vi "FPGA_fast cycles-5.vi"() -> ()   [LabVIEW 2013]
uses:
  FPGA_run-states.ctl
  <vilib>/rvi/Emulation/niFpgaSctlEmulationGetInTimedLoop.vi
  <vilib>/rvi/Emulation/niFpgaEmulationReportErrorSimple.vi
  <vilib>/rvi/Emulation/niFpgaGetClockAttributes.vi
  <vilib>/rvi/Emulation/niFpgaCriticalErrorInLSC.vi
  <vilib>/rvi/eio/common/nirviEmuTemplateMethod_errors.vi
  <vilib>/rvi/FIFO/Fifo_Resource/nirvififoEmulationReadFpgaImpl.vi
  <vilib>/rvi/DataTransferAndStorage/Container/Common/niFpgaContainerGetUniqueNameForEmu.vi
  <vilib>/rvi/Emulation/niFpgaProcessEmulError.vi
  <vilib>/rvi/Memory/Memory_Emulation/nirvimemoryEmulation.vi
  <vilib>/rvi/Memory/Memory_Emulation/nirvimemoryFastEmulation.vi
  <vilib>/rvi/Memory/Memory_Emulation/niFpgaMemoryEmulationCacheClearOnFirstRun.vi
  <vilib>/rvi/Memory/Memory_Emulation/nirvimemoryEmulationManagerCache_MakeExclusive.vi
  <vilib>/rvi/Memory/Memory_Emulation/niFpgaMemoryEmulationValidateCache.vi
  <vilib>/rvi/Memory/Memory_Emulation/nirvimemoryEmulationManagerCache_ReleaseExclusive.vi
  <vilib>/rvi/Memory/Memory_Emulation/nirvimemoryEmulationManagerCache_InsertValue.vi
  <vilib>/Utility/error.llb/Clear Errors.vi
  <vilib>/rvi/Memory/Memory_Emulation/nirvimemoryEmulationManagerCache_SetValue.vi
  <vilib>/rvi/Emulation/niFpgaSctlEmulationResourceMgr.vi
  <vilib>/rvi/Memory/Memory_Emulation/nirvimemoryEmulationManagerCache_GetValue.vi
  <vilib>/rvi/Memory/Memory_Emulation/nirvimemoryFastEmulationFpgaImpl.vi
  <instcachedir>/0/nirvimemoryFastEmulationFpgaImpl_5FBAB50466BC4C939F684F8805638BFC.lvgen/nirvimemoryFastEmulationFpgaImpl_5FBAB50466BC4C939F684F8805638BFC_004.vi
  <vilib>/rvi/FIFO/Fifo_Resource/nirvififoEmulationWriteFpgaImpl.vi
  <vilib>/eio/EIONode/EIONode.xnode
  <vilib>/rvi/DataTransferAndStorage/Container/XNode/niFpgaContainer.xnode
  <vilib>/rvi/FIFO/Fifo_Resource/nirvififoEmulationRead.vi
  <vilib>/rvi/FIFO/Fifo_Resource/nirvififoEmulationWrite.vi
panel:
  in  "start ind":u32
  out "stopped":bool=TRUE
  out "ramp":bool
  out "trigDAC":bool
  in  "order in":u64=360850920143060992
  in  "get order":bool
  in  "trig dur (us)":u16=100
  in  "us per DAC":u32=1000
  out "gen trig":bool
  in  "Stop seq":bool=TRUE
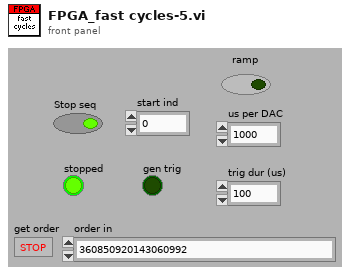
[diagram p1: front panel]
types:
  T1 = typedef "FPGA_run-states.ctl" = enum16{"stopped", "check", "reserve", "run", "release"}
  T2 = cluster{"Boolean array[0]":bool, "Boolean array[1]":bool, "Boolean array[2]":bool, "Boolean array[3]":bool, "Boolean array[4]":bool, "Boolean array[5]":bool, "Boolean array[6]":bool, "Boolean array[7]":bool, "Boolean array[8]":bool, "Boolean array[9]":bool}
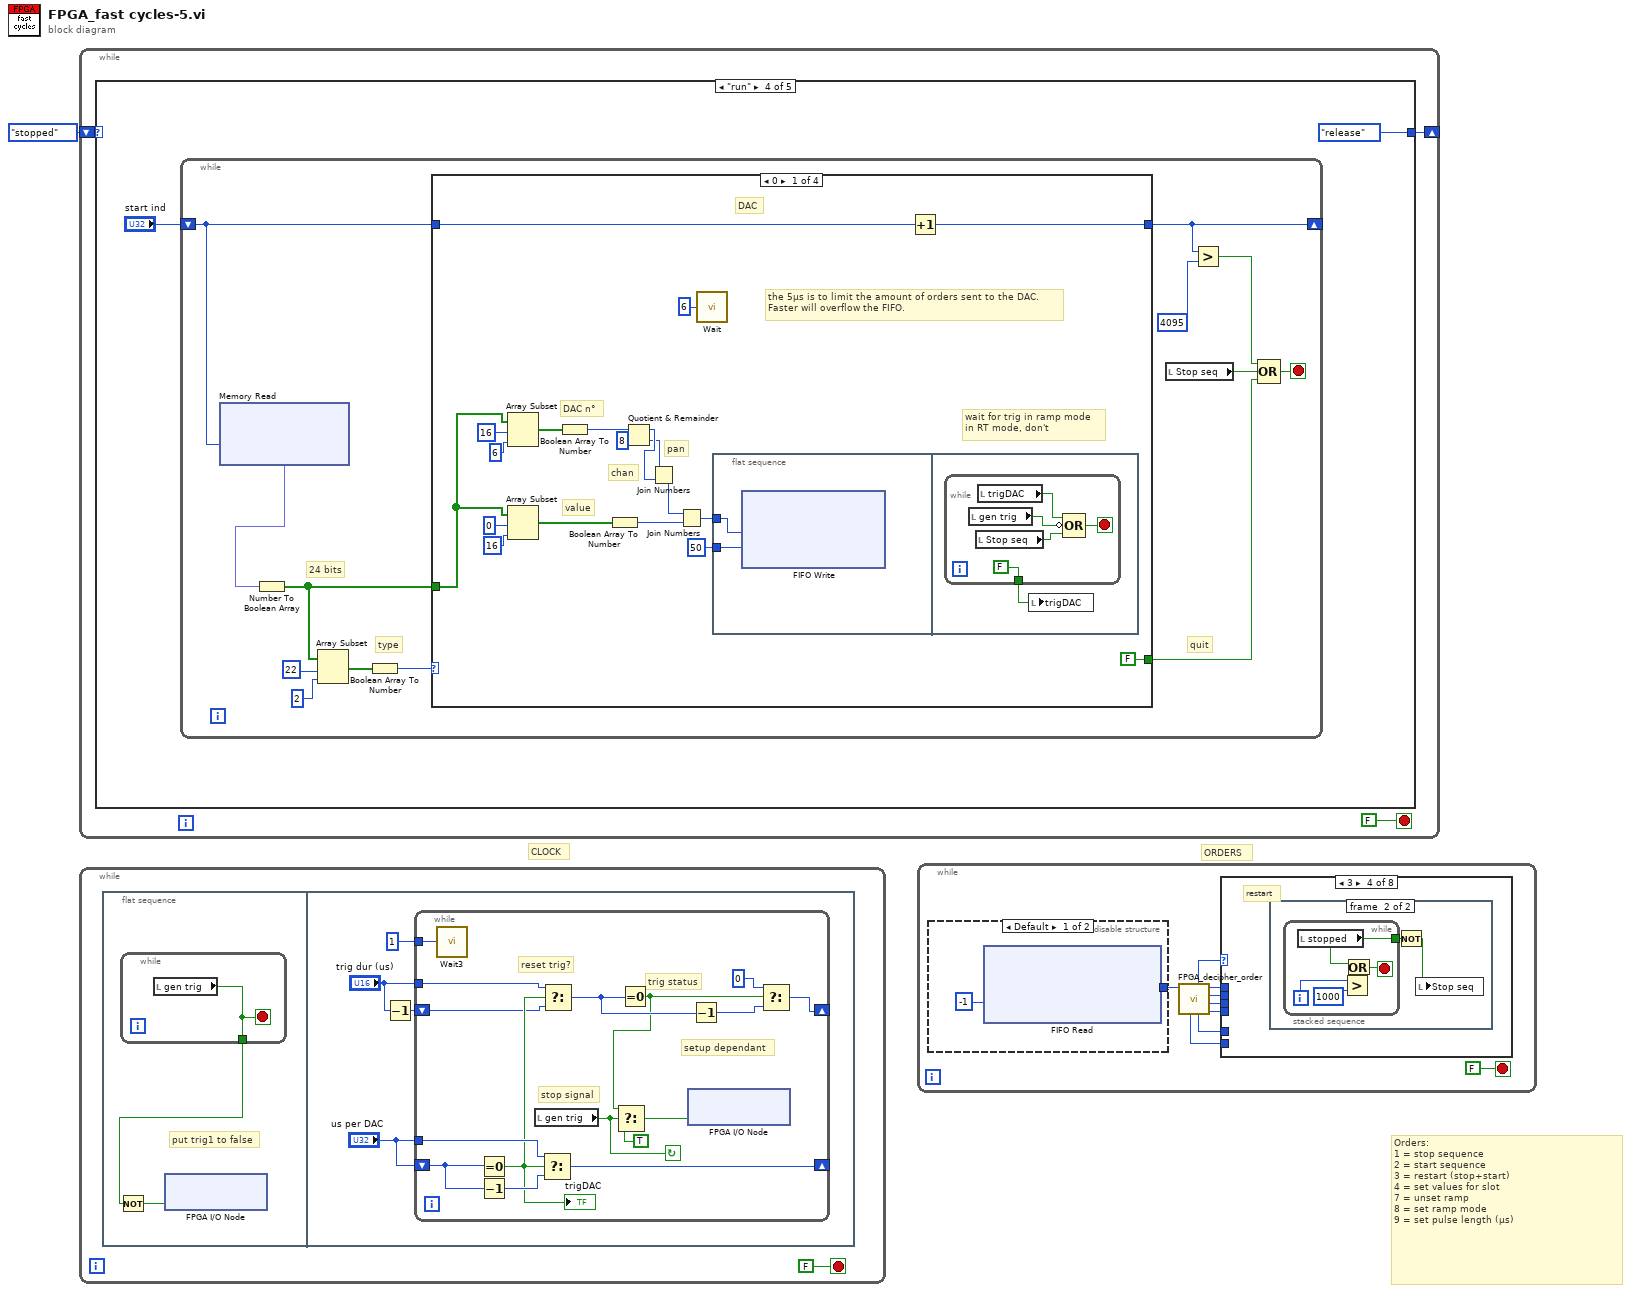
[diagram p0: block diagram]
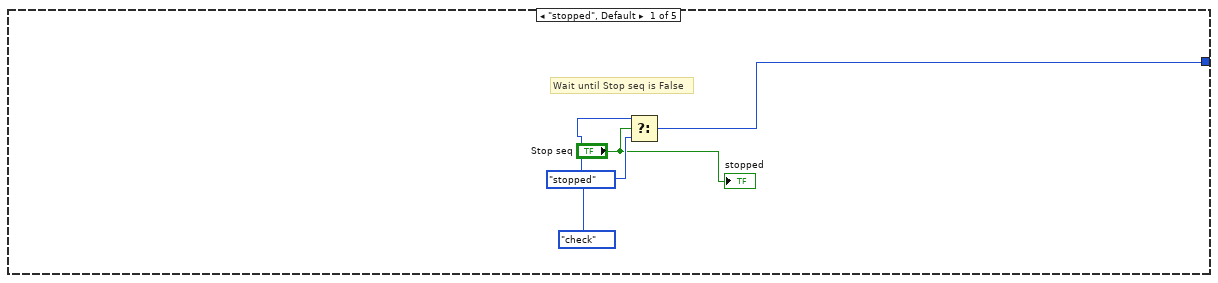
[diagram p2: hidden frame]
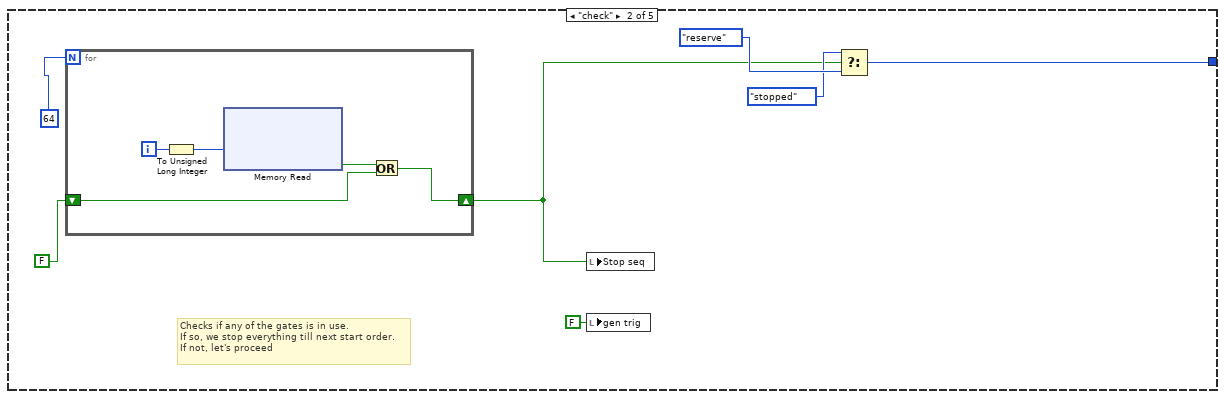
[diagram p3: hidden frame]
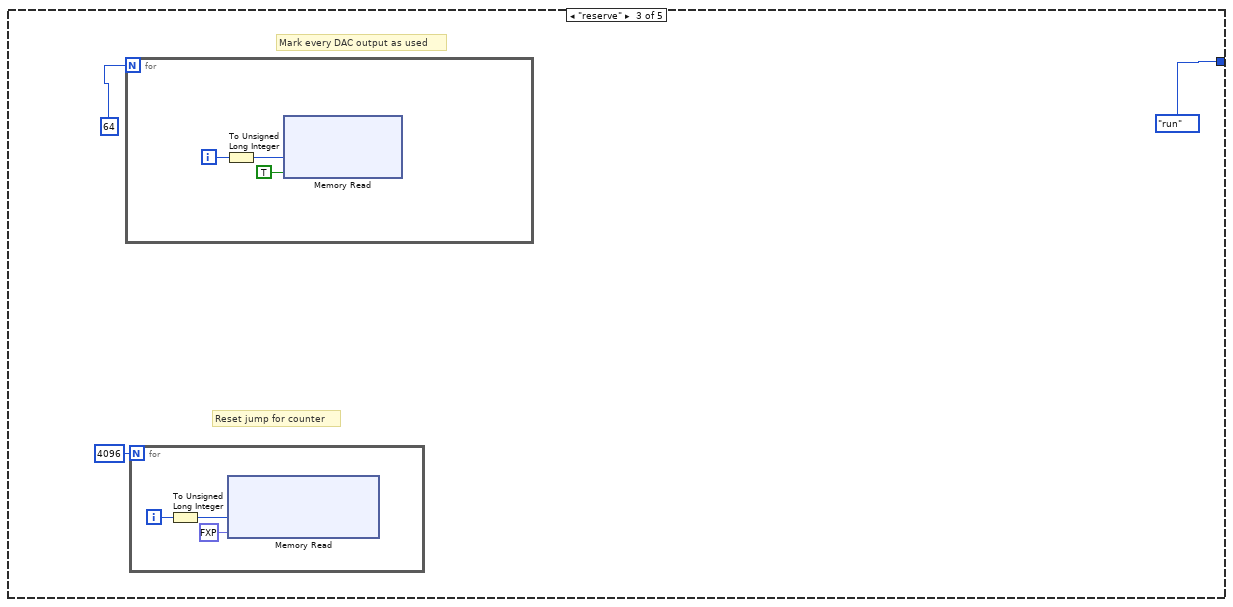
[diagram p4: hidden frame]
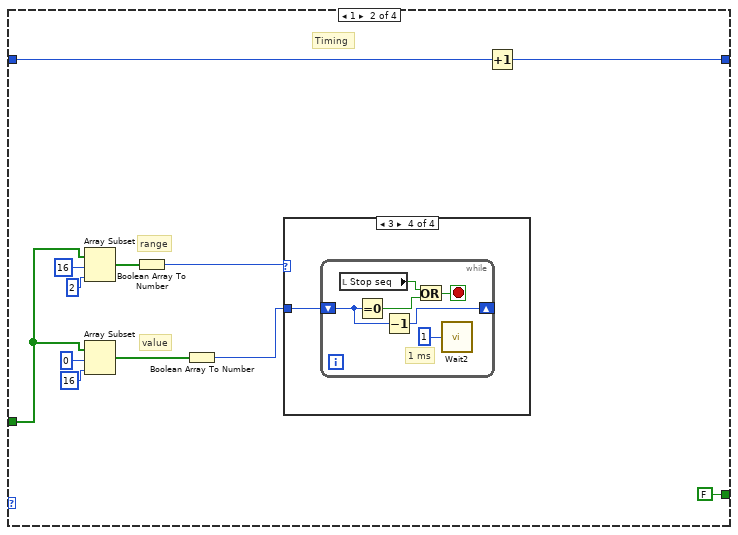
[diagram p5: hidden frame]
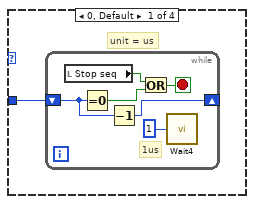
[diagram p6: hidden frame]
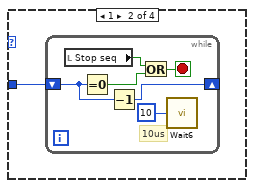
[diagram p7: hidden frame]
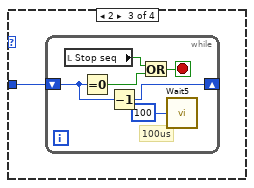
[diagram p8: hidden frame]
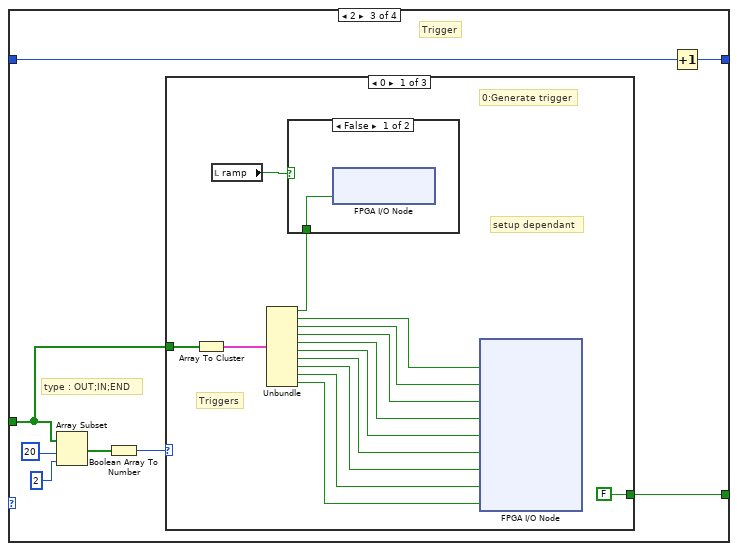
[diagram p9: hidden frame]
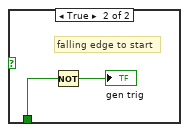
[diagram p10: hidden frame]
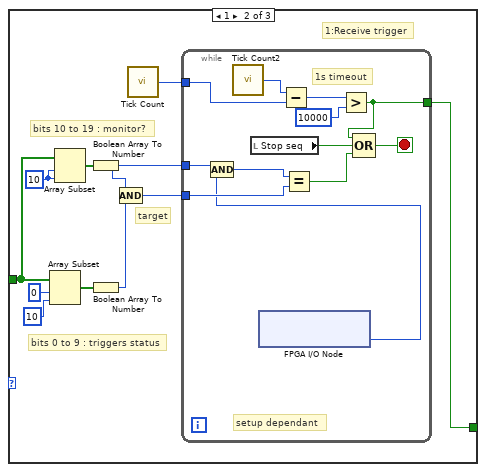
[diagram p11: hidden frame]
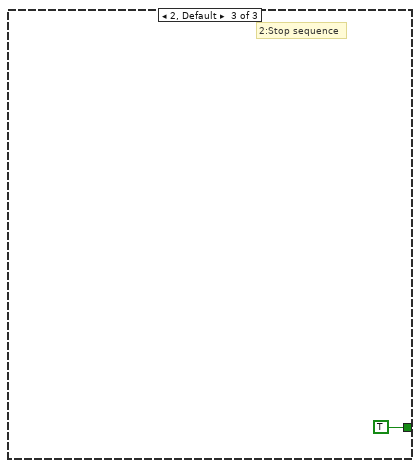
[diagram p12: hidden frame]
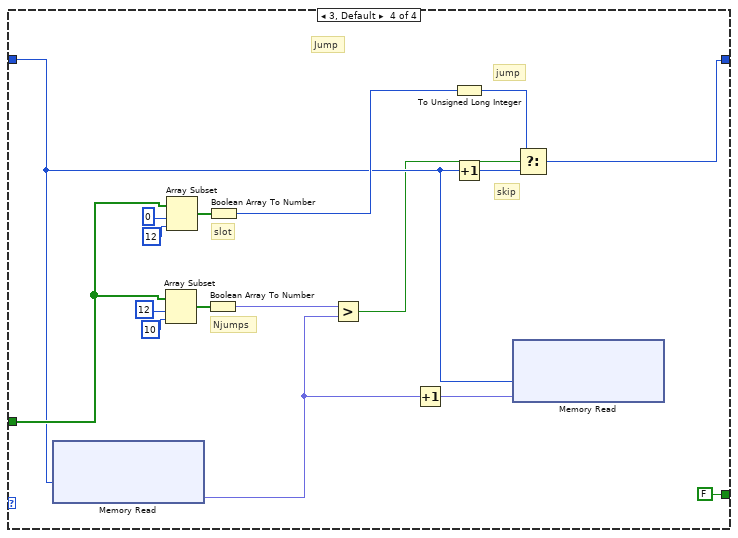
[diagram p13: hidden frame]
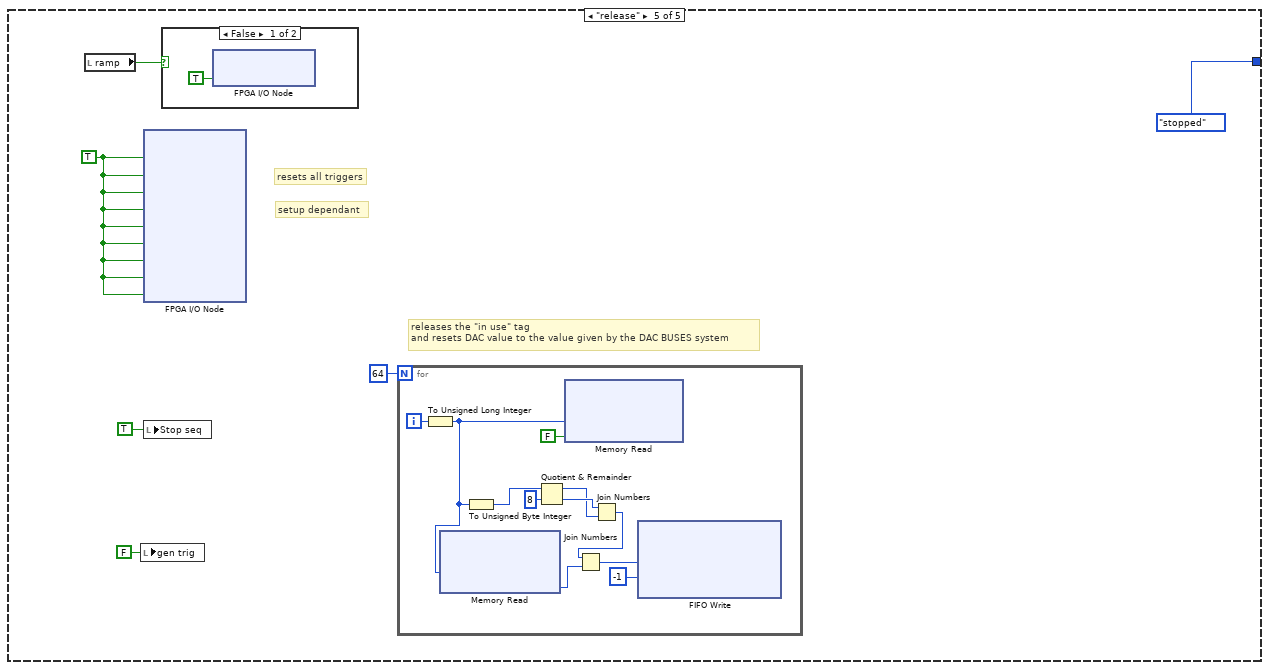
[diagram p14: hidden frame]
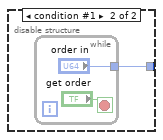
[diagram p16: hidden frame]
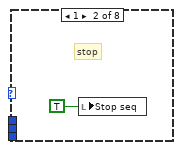
[diagram p18: hidden frame]
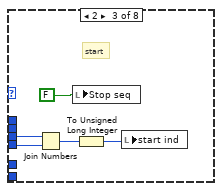
[diagram p19: hidden frame]
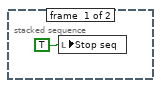
[diagram p20: hidden frame]
diagram:
  # "ORDERS"
  # "CLOCK"
  # "Orders:\n1 = stop sequence\n2 = start sequence\n3 = restart (stop+start)\n4 = set values for slot\n7 = unset ramp\n8 = set ramp mode\n9 = set pulse length (µs)"
  n1 = while {
    shift-right: [w2] -> _
    shift-left: FPGA_run-states."stopped" ("run states") -> [w3]
    stop <- FALSE stop-if-true
    n2 = case shown="\"run\"" w3 {
      tunnel: [w6 w10 FPGA_run-states."run" ("run states") FPGA_run-states."release" ("run states") FPGA_run-states."stopped" ("run states")] -> w2
      frame "stopped", Default {
        # "Wait until Stop seq is False"
        n3 = Select(t=FPGA_run-states."stopped" ("run states"), s="Stop seq", f=FPGA_run-states."check" ("run states")) -> (s? t:f=w6:T1)
        "stopped" <- "Stop seq"
      }
      frame "check" {
        # "Checks if any of the gates is in use.\nIf so, we stop everything till next start order.\nIf not, let's proceed"
        n4 = for {
          N: 64 -> [_]
          shift-right: [w16] -> w11
          shift-left: FALSE ("Data") -> [w19]
          i -> [w18]
          n5 = To Unsigned Long Integer(number=w18) -> (unsigned 32bit integer=w17:u32)
          n6 = xnode ("Memory Read")("Address"=w17) -> ("Data"=w20:bool)  [unwired: 1 in, 1 out]
          n7 = Or(x=w20, y=w19) -> (x .or. y?=w16:bool)
        }
        n8 = local write "Stop seq"(w11) -> ()
        n9 = local write "gen trig"(FALSE ("gen trig")) -> ()
        n10 = Select(t=FPGA_run-states."stopped" ("run states"), s=w11, f=FPGA_run-states."reserve" ("run states")) -> (s? t:f=w10:T1)
      }
      frame "reserve" {
        # "Reset jump for counter"
        # "Mark every DAC output as used"
        n11 = for {
          N: 64 -> [_]
          i -> [w29]
          n12 = To Unsigned Long Integer(number=w29) -> (unsigned 32bit integer=w28:u32)
          n13 = xnode ("Memory Read")("Address"=w28, "Data"=TRUE) -> ()  [unwired: 1 in, 1 out]
        }
        n14 = for {
          N: 4096 -> [_]
          i -> [w26]
          n15 = To Unsigned Long Integer(number=w26) -> (unsigned 32bit integer=w25:u32)
          n16 = xnode ("Memory Read")("Address"=w25, "Data"=fxp<+,10,10> 0.0) -> ()  [unwired: 1 in, 1 out]
        }
      }
      frame "run" {
        n17 = while {
          shift-right: [w38] -> _
          shift-left: "start ind" -> [w40]
          stop <- w35 stop-if-true
          # "24 bits"
          # "quit"
          # "type"
          n18 = xnode ("Memory Read")("Address"=w40) -> ("Data"=w33:fxp<+,24,24>)  [unwired: 1 in, 1 out]
          n19 = Number To Boolean Array(number=w33) -> (Boolean array=w32:bool[])
          n20 = Array Subset(array=w32, index=22 ("length"), length=2 ("index")) -> (w42:bool[])
          n21 = Boolean Array To Number(Boolean array=w42) -> (number=w41:u16)
          n22 = case shown="0" w41 {
            tunnel: w40 -> [w62 w83 w114 w163]
            tunnel: [w60 w82 w119 w169] -> w38
            tunnel: w32 -> [w45 w74 w115 w167]
            tunnel: [FALSE ("[15]") FALSE ("[15]") w112 FALSE ("[15]")] -> w34
            frame 0 {
              # "chan"
              # "pan"
              # "DAC n°"
              # "value"
              # "wait for trig in ramp mode\nin RT mode, don't"
              # "DAC"
              # "the 5µs is to limit the amount of orders sent to the DAC.\nFaster will overflow the FIFO."
              n23 = Array Subset(array=w45, index=16 ("length"), length=6 ("index")) -> (w52:bool[])
              n24 = Array Subset(array=w45, index=0 ("length"), length=16 ("index")) -> (w47:bool[])
              n25 = Boolean Array To Number(Boolean array=w52) -> (number=w46:u8)
              n26 = Boolean Array To Number(Boolean array=w47) -> (number=w61:u16)
              n27 = Quotient & Remainder(x=w46, y=u8 8) -> (x-y*floor(x/y)=w56:u8, floor(x/y)=w55:u8)
              n28 = Join Numbers(hi=w55, lo=w56) -> ((hi.lo)=w54:u16)
              n29 = Join Numbers(hi=w54, lo=w61) -> ((hi.lo)=w59:u32)
              n30 = call "Wait"("Count(uSec)"=u8 6) -> ()  [unwired: 1 out]
              n31 = flat-sequence {
                tunnel: w59 -> [w65]
                tunnel: 50 ("Timeout") -> [w64]
                frame #0 {
                  n32 = xnode ("FIFO Write")("Element"=w65, "Timeout"=w64) -> ()  [unwired: 1 in, 2 out]
                }
                frame #1 {
                  n33 = while {
                    tunnel: [FALSE ("Stop seq 3")] -> w66
                    stop <- w68 stop-if-true
                    n34 = local read "gen trig"() -> (w70:bool)
                    n35 = local read "Stop seq"() -> (w71:bool)
                    n36 = local read "trigDAC"() -> (w69:bool)
                    n37 = Compound Arithmetic op=OR(w69, invert w70, w71) -> (w68:bool)
                  }
                  n38 = local write "trigDAC"(w66) -> ()
                }
              }
              n39 = Increment(x=w62) -> (x+1=w60:u32)
            }
            frame 1 {
              # "range"
              # "value"
              # "Timing"
              n40 = Array Subset(array=w74, index=16 ("length"), length=2 ("index")) -> (w80:bool[])
              n41 = Array Subset(array=w74, index=0 ("length"), length=16 ("index")) -> (w75:bool[])
              n42 = Boolean Array To Number(Boolean array=w80) -> (number=w73:u8)
              n43 = Boolean Array To Number(Boolean array=w75) -> (number=w72:u16)
              n44 = case shown="3" w73 {
                tunnel: w72 -> [w84 w91 w98 w105]
                frame 0, Default {
                  # "unit = us"
                  n45 = while {
                    shift-right: [w85] -> _
                    shift-left: w84 -> [w86]
                    stop <- w90 stop-if-true
                    # "1us"
                    n46 = local read "Stop seq"() -> (w87:bool)
                    n47 = Equal To 0?(x=w86) -> (x = 0?=w88:bool)
                    n48 = Decrement ("Décrémenter")(x=w86) -> (x-1=w85:u16)
                    n49 = Or(x=w87, y=w88) -> (x .or. y?=w90:bool)
                    n50 = call "Wait4"("Count(uSec)"=u8 1) -> ()  [unwired: 1 out]
                  }
                }
                frame 1 {
                  n51 = while {
                    shift-right: [w92] -> _
                    shift-left: w91 -> [w93]
                    stop <- w97 stop-if-true
                    # "10us"
                    n52 = local read "Stop seq"() -> (w94:bool)
                    n53 = Equal To 0?(x=w93) -> (x = 0?=w95:bool)
                    n54 = Decrement ("Décrémenter")(x=w93) -> (x-1=w92:u16)
                    n55 = Or(x=w94, y=w95) -> (x .or. y?=w97:bool)
                    n56 = call "Wait6"("Count(uSec)"=u8 10) -> ()  [unwired: 1 out]
                  }
                }
                frame 2 {
                  n57 = while {
                    shift-right: [w99] -> _
                    shift-left: w98 -> [w100]
                    stop <- w104 stop-if-true
                    # "100us"
                    n58 = local read "Stop seq"() -> (w101:bool)
                    n59 = Equal To 0?(x=w100) -> (x = 0?=w102:bool)
                    n60 = Decrement ("Décrémenter")(x=w100) -> (x-1=w99:u16)
                    n61 = Or(x=w101, y=w102) -> (x .or. y?=w104:bool)
                    n62 = call "Wait5"("Count(uSec)"=u8 100) -> ()  [unwired: 1 out]
                  }
                }
                frame 3 {
                  n63 = while {
                    shift-right: [w106] -> _
                    shift-left: w105 -> [w107]
                    stop <- w111 stop-if-true
                    # "1 ms"
                    n64 = local read "Stop seq"() -> (w108:bool)
                    n65 = Equal To 0?(x=w107) -> (x = 0?=w109:bool)
                    n66 = Decrement ("Décrémenter")(x=w107) -> (x-1=w106:u16)
                    n67 = Or(x=w108, y=w109) -> (x .or. y?=w111:bool)
                    n68 = call "Wait2"("Count(mSec)"=u8 1 ("Count(uSec)")) -> ()  [unwired: 1 out]
                  }
                }
              }
              n69 = Increment(x=w83) -> (x+1=w82:u32)
            }
            frame 2 {
              # "type : OUT;IN;END"
              # "Trigger"
              n70 = Array Subset(array=w115, index=20 ("length"), length=2 ("index")) -> (w118:bool[])
              n71 = Boolean Array To Number(Boolean array=w118) -> (number=w113:u16)
              n72 = case shown="0" w113 {
                tunnel: w115 -> [w130 w145 _]
                tunnel: [FALSE ("[15]") w137 TRUE ("[15]")] -> w112
                frame 0 {
                  # "0:Generate trigger"
                  # "setup dependant"
                  # "Triggers"
                  n73 = Array To Cluster(array=w130) -> (cluster=w133:T2)
                  n74 = local read "ramp"() -> (w131:bool)
                  n75 = Unbundle(w133) -> ("Boolean array[0]"=w132:bool, "Boolean array[1]"=w128:bool, "Boolean array[2]"=w127:bool, "Boolean array[3]"=w126:bool, "Boolean array[4]"=w125:bool, "Boolean array[5]"=w124:bool, "Boolean array[6]"=w123:bool, "Boolean array[7]"=w122:bool, "Boolean array[8]"=w121:bool, "Boolean array[9]"=w120:bool)
                  n76 = case shown="False" w131 {
                    tunnel: w132 -> [w134 w136]
                    frame False {
                      n77 = xnode "FPGA I/O Node"("Port0/DIO0"=w134) -> ()  [unwired: 1 in, 1 out]
                    }
                    frame True {
                      # "falling edge to start"
                      n78 = Not(x=w136) -> (.not. x?=→"gen trig":bool)
                    }
                  }
                  n79 = xnode "FPGA I/O Node"("Port0/DIO1"=w128, "Port0/DIO2"=w127, "Port0/DIO3"=w126, "Port0/DIO4"=w125, "Port0/DIO5"=w124, "Port0/DIO6"=w123, "Port0/DIO7"=w122, "Port0/DIO8"=w121, "Port0/DIO9"=w120) -> ()  [unwired: 9 in, 9 out]
                }
                frame 1 {
                  w147 = 10 ("index")
                  # "target"
                  # "bits 10 to 19 : monitor?"
                  # "1:Receive trigger"
                  # "bits 0 to 9 : triggers status"
                  n80 = Array Subset(array=w145, index=0, length=10 ("index")) -> (w143:bool[])
                  n81 = Array Subset(array=w145, index=w147, length=w147) -> (w142:bool[])
                  n82 = Boolean Array To Number(Boolean array=w142) -> (number=w141:u16)
                  n83 = Boolean Array To Number(Boolean array=w143) -> (number=w139:u16)
                  n84 = Compound Arithmetic op=AND(w141, w139) -> (w140:u16)
                  n85 = call "Tick Count"() -> ("Tick Count(mSec)"=w138:u32)
                  n86 = while {
                    tunnel: w141 -> [w159]
                    tunnel: w140 -> [w157]
                    tunnel: w138 -> [w153]
                    tunnel: [w149] -> w137
                    stop <- w150 stop-if-true
                    # "1s timeout"
                    # "setup dependant"
                    n87 = call "Tick Count2"() -> ("Tick Count(mSec)"=w156:u32)
                    n88 = local read "Stop seq"() -> (w152:bool)
                    n89 = xnode "FPGA I/O Node"() -> ("Port8/DIO9:0"=w148:u16)  [unwired: 1 in, 1 out]
                    n90 = Compound Arithmetic op=AND(w159, w148) -> (w158:u16)
                    n91 = Subtract(x=w156, y=w153) -> (x-y=w154:u32)
                    n92 = Equal?(x=w158, y=w157) -> (x = y?=w151:bool)
                    n93 = Greater?(x=w154, y=u32 10000 ("Tick Count(mSec)")) -> (0:w149:bool)
                    n94 = Compound Arithmetic op=OR(w149, w152, w151) -> (w150:bool)
                  }
                }
                frame 2, Default {
                  # "2:Stop sequence"
                }
              }
              n95 = Increment(x=w114) -> (x+1=w119:u32)
            }
            frame 3, Default {
              # "skip"
              # "jump"
              # "Njumps"
              # "slot"
              # "Jump"
              n96 = xnode ("Memory Read")("Address"=w163) -> ("Data"=w161:fxp<+,10,10>)  [unwired: 1 in, 1 out]
              n97 = Array Subset(array=w167, index=12 ("length"), length=10 ("index")) -> (w175:bool[])
              n98 = Array Subset(array=w167, index=0 ("length"), length=12 ("index")) -> (w168:bool[])
              n99 = Boolean Array To Number(Boolean array=w175) -> (number=w165:fxp<+,10,10>)
              n100 = Boolean Array To Number(Boolean array=w168) -> (number=w172:u16)
              n101 = Greater?(x=w165, y=w161) -> (0:w162:bool)
              n102 = Increment(x=w161) -> (x+1=w164:fxp<+,11,11>)
              n103 = To Unsigned Long Integer(number=w172) -> (unsigned 32bit integer=w170:u32)
              n104 = Increment(x=w163) -> (x+1=w171:u32)
              n105 = xnode ("Memory Read")("Address"=w163, "Data"=w164) -> ()  [unwired: 1 in, 1 out]
              n106 = Select(t=w170, s=w162, f=w171) -> (s? t:f=w169:u32)
            }
          }
          n107 = local read "Stop seq"() -> (w37:bool)
          n108 = Greater?(x=w38, y=u32 4095) -> (0:w36:bool)
          n109 = Compound Arithmetic op=OR(w36, w37, w34) -> (w35:bool)
        }
      }
      frame "release" {
        w178 = TRUE ("Port9/DIO1")
        # "setup dependant"
        # "resets all triggers"
        # "releases the \"in use\" tag\nand resets DAC value to the value given by the DAC BUSES system"
        n110 = local read "ramp"() -> (w179:bool)
        n111 = local write "gen trig"(FALSE ("ramp")) -> ()
        n112 = xnode "FPGA I/O Node"("Port0/DIO1"=w178, "Port0/DIO2"=w178, "Port0/DIO3"=w178, "Port0/DIO4"=w178, "Port0/DIO5"=w178, "Port0/DIO6"=w178, "Port0/DIO7"=w178, "Port0/DIO8"=w178, "Port0/DIO9"=w178) -> ()  [unwired: 9 in, 9 out]
        n113 = local write "Stop seq"(TRUE ("Boolean array[15]")) -> ()
        n114 = case shown="False" w179 {
          frame False {
            n115 = xnode "FPGA I/O Node"("Port0/DIO0"=TRUE ("Port9/DIO0")) -> ()  [unwired: 1 in, 1 out]
          }
          frame True {
          }
        }
        n116 = for {
          N: 64 -> [_]
          i -> [w191]
          n117 = To Unsigned Long Integer(number=w191) -> (unsigned 32bit integer=w186:u32)
          n118 = xnode ("Memory Read")("Address"=w186) -> ("Data"=w192:u16)  [unwired: 1 in, 1 out]
          n119 = To Unsigned Byte Integer(number=w186) -> (unsigned 8bit integer=w187:u8)
          n120 = Quotient & Remainder(x=w187, y=u8 8) -> (x-y*floor(x/y)=w188:u8, floor(x/y)=w189:u8)
          n121 = xnode ("Memory Read")("Address"=w186, "Data"=FALSE) -> ()  [unwired: 1 in, 1 out]
          n122 = Join Numbers(hi=w189, lo=w188) -> ((hi.lo)=w185:u16)
          n123 = Join Numbers(hi=w185, lo=w192) -> ((hi.lo)=w193:u32)
          n124 = xnode ("FIFO Write")("Element"=w193, "Timeout"=-1) -> ()  [unwired: 1 in, 2 out]
        }
      }
    }
  }
  n125 = while {
    stop <- FALSE stop-if-true
    n126 = flat-sequence {
      frame #0 {
        # "put trig1 to false"
        n127 = while {
          tunnel: [w199] -> w198
          stop <- w199 stop-if-true
          n128 = local read "gen trig"() -> (w199:bool)
        }
        n129 = Not(x=w198) -> (.not. x?=w197:bool)
        n130 = xnode "FPGA I/O Node"("Port0/DIO0"=w197) -> ()  [unwired: 1 in, 1 out]
      }
      frame #1 {
        n131 = Decrement(x="trig dur (us)") -> (x-1=w200:u16)
        n132 = while {
          tunnel: u8 1 ("Count(Ticks)") -> [w219]
          tunnel: "trig dur (us)" -> [w213]
          tunnel: "us per DAC" -> [w216]
          shift-right: [w218] -> _
          shift-left: "us per DAC" -> [w215]
          shift-right: [w208] -> _
          shift-left: w200 -> [w212]
          stop <- w205 continue-if-true
          # "stop signal"
          # "setup dependant"
          # "trig status"
          # "reset trig?"
          n133 = call "Wait3"("Count(uSec)"=w219) -> ()  [unwired: 1 out]
          n134 = Equal To 0?(x=w215) -> (x = 0?=w214:bool)
          "trigDAC" <- w214
          n135 = Decrement(x=w215) -> (x-1=w217:u32)
          n136 = local read "gen trig"() -> (w205:bool)
          n137 = Select(t=w216, s=w214, f=w217) -> (s? t:f=w218:u32)
          n138 = Select(t=w213, s=w214, f=w212) -> (s? t:f=w209:u16)
          n139 = Equal To 0?(x=w209) -> (x = 0?=w207:bool)
          n140 = Select(t=w207, s=w205, f=TRUE) -> (s? t:f=w204:bool)
          n141 = xnode "FPGA I/O Node"("Port0/DIO0"=w204) -> ()  [unwired: 1 in, 1 out]
          n142 = Decrement(x=w209) -> (x-1=w211:u16)
          n143 = Select(t=u16 0, s=w207, f=w211) -> (s? t:f=w208:u16)
        }
      }
    }
  }
  n144 = while {
    stop <- FALSE stop-if-true
    n145 = disable-structure shown="Default" {
      disable-tunnel: [w229 w231] -> w227
      frame condition #0 (active) {
        n146 = xnode ("FIFO Read")("Timeout"=-1) -> ("Element"=w229:u64)  [unwired: 1 in, 2 out]
      }
      frame condition #1 {
        n147 = while {
          tunnel: ["order in"] -> w231
          stop <- "get order" stop-if-true
        }
      }
    }
    n148 = call "FPGA_decipher_order.vi"("order in"=w227) -> ("data 1"=w225:u8, "data 2"=w224:u8, "data 3"=w222:u8, "data 4"=w223:u8, "RFU 2"=w220:u8, "order out"=w226:u8, "RFU 1"=w221:u8)  [unwired: 3 in, 1 out]
    n149 = case shown="3" w226 {
      tunnel: w225 -> [_ _ w236 _ w259 _ w265 w271]
      tunnel: w224 -> [_ _ w237 _ w258 _ w266 w270]
      tunnel: w223 -> [_ _ _ _ w256 _ w268 _]
      tunnel: w222 -> [_ _ _ _ w257 _ w267 _]
      tunnel: w221 -> [_ _ _ _ w250 _ _ _]
      tunnel: w220 -> [_ _ _ _ w251 _ _ _]
      frame 0, Default {
      }
      frame 1 {
        # "stop"
        n150 = local write "Stop seq"(TRUE ("Stop seq")) -> ()
      }
      frame 2 {
        # "start"
        n151 = Join Numbers(hi=w237, lo=w236) -> ((hi.lo)=w238:u16)
        n152 = local write "Stop seq"(FALSE ("Stop seq")) -> ()
        n153 = To Unsigned Long Integer(number=w238) -> (unsigned 32bit integer=w235:u32)
        n154 = local write "start ind"(w235) -> ()
      }
      frame 3 {
        # "restart"
        n155 = stacked-sequence {
          frame #0 {
            n156 = local write "Stop seq"(TRUE ("Stop seq")) -> ()
          }
          frame #1 {
            n157 = while {
              tunnel: [w243] -> w242
              i -> [w247]
              stop <- w244 stop-if-true
              n158 = local read "stopped"() -> (w243:bool)
              n159 = Greater?(x=w247, y=1000) -> (0:w245:bool)
              n160 = Or(x=w243, y=w245) -> (x .or. y?=w244:bool)
            }
            n161 = Not(x=w242) -> (.not. x?=w241:bool)
            n162 = local write "Stop seq"(w241) -> ()
          }
        }
      }
      frame 4 {
        # "update slot"
        n163 = Join Numbers(hi=w256, lo=w257) -> ((hi.lo)=w254:u16)
        n164 = Join Numbers(hi=w258, lo=w259) -> ((hi.lo)=w255:u16)
        n165 = Join Numbers(hi=w251, lo=w250) -> ((hi.lo)=w249:u16)
        n166 = Join Numbers(hi=w254, lo=w255) -> ((hi.lo)=w253:u32)
        n167 = To Unsigned Long Integer(number=w249) -> (unsigned 32bit integer=w248:u32)
        n168 = To Fixed-Point(number=w253) -> (fixed-point=w252:fxp<+,24,24>)  [unwired: 1 in]
        n169 = xnode ("Memory Write")("Address"=w248, "Data"=w252) -> ()  [unwired: 1 in, 1 out]
      }
      frame 7 {
        w260 = FALSE ("trigDAC")
        # "disable ramp mode"
        n170 = local write "gen trig"(w260) -> ()
        "ramp" <- w260
      }
      frame 8 {
        # "set ramp"
        n171 = Join Numbers(hi=w268, lo=w267) -> ((hi.lo)=w264:u16)
        n172 = Join Numbers(hi=w266, lo=w265) -> ((hi.lo)=w263:u16)
        n173 = Join Numbers(hi=w264, lo=w263) -> ((hi.lo)=w262:u32)
        n174 = local write "us per DAC"(w262) -> ()
        n175 = local write "ramp"(TRUE ("ramp")) -> ()
      }
      frame 9 {
        # "set the length of the trigger"
        n176 = Join Numbers(hi=w270, lo=w271) -> ((hi.lo)=w269:u16)
        n177 = local write "trig dur (us)"(w269) -> ()
      }
    }
  }
